vi "CIEdgesProps.vi"(5 "task in":refnum<k24>, 7 "error in (no error)":errorcluster) -> (0 "task out":refnum<k24>, 1 "Edge":i32, 2 "InitialCount":u32, 3 "error out":errorcluster, 4 "Direction":i32, 6 "Gate Function":i32)   [LabVIEW 2010]
uses:
  C:/Program Files/National Instruments/LabVIEW 2010/vi.lib/ULx/ULx_LV.dll
  Program Files/National Instruments/LabVIEW 2010/vi.lib/ULx/ULx_LV.dll
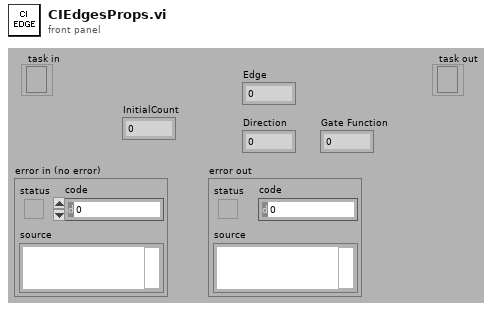
[diagram p1: front panel]
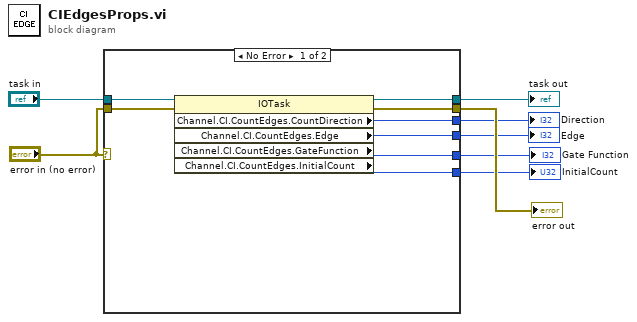
[diagram p0: block diagram]
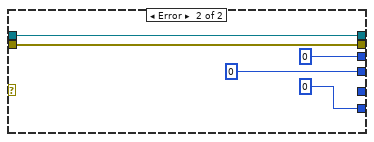
[diagram p2: hidden frame]
diagram:
  n1 = case shown="No Error" "error in (no error)" {
    tunnel: "task in" -> [w16 w21]
    tunnel: "error in (no error)" -> [w15 w20]
    tunnel: [w13 w21] -> w7
    tunnel: [w14 w20] -> w6
    tunnel: [w11 0 ("Channel.AI.Temp.Units")] -> w4
    tunnel: [w9 u32 0 ("Channel.CI.CountEdges.InitialCount")] -> w3
    tunnel: [w12 0 ("Channel.CI.CountEdges.CountDirection")] -> w2
    tunnel: [w10 _] -> w1
    frame No Error {
      n2 = property class="IOTask"(reference=w16, error in=w15) -> (reference out=w13:refnum<k24>, error out=w14:errorcluster, "Channel.CI.CountEdges.CountDirection"=w12:i32, "Channel.CI.CountEdges.Edge"=w11:i32, "Channel.CI.CountEdges.GateFunction"=w10:i32, "Channel.CI.CountEdges.InitialCount"=w9:u32)
    }
    frame Error {
    }
  }
  "task out" <- w7
  "error out" <- w6
  "Edge" <- w4
  "InitialCount" <- w3
  "Direction" <- w2
  "Gate Function" <- w1
